vi "Configure Multi Eval Meas List Segment Modulation.vi"(0 "VISA resource name":refnum<visa-resource-name>, 1 "Enable (Off)":bool, 2 "MERR Enable (Off)":bool, 3 "Inband Emission Enable (Off)":bool, 5 "Instance (1)":T1=1, 7 "Segment (1)":i32=1, 9 "Statistics (20)":i32=20, 11 "error in (no error)":errorcluster, 12 "EVM Enable (Off)":bool, 13 "PERR Enable (Off)":bool, 14 "EQ Spectrum Flatness Enable (Off)":bool) -> (4 "VISA resource name out":refnum<visa-resource-name>, 15 "error out":errorcluster)   [LabVIEW 2020, in "Rohde&Schwarz CMWXP NR FR1 Measurement.lvlib"]
doc: "Defines settings for modulation measurements in list mode for segment <no>.\n\nAttribute:\nRSCMWXPNRFR1M_ATTR_MULTI_EVAL_MEAS_LIST_SEGMENT_MODULATION\n\nRemote-control command:\nCONFigure:NRSub:MEAS<i>:MEValuation:LIST:SEGMent<no>:MODulation"
uses:
  <instrlib>/Rohde&Schwarz CMWXP NR FR1 Measurement/Rohde&Schwarz CMWXP NR FR1 Measurement.lvlib
  <instrlib>/Rohde&Schwarz CMWXP NR FR1 Measurement/Private/_Instance.ctl
  <instrlib>/Rohde&Schwarz CMWXP NR FR1 Measurement/Private/rsidr_core.llb/rsidr_core.lvlib
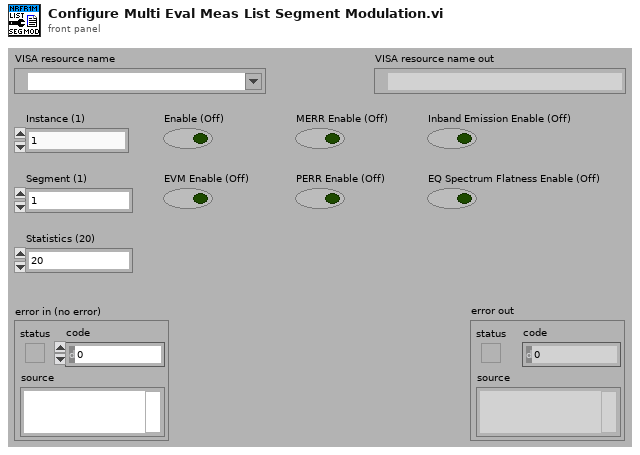
[diagram p1: front panel]
types:
  T1 = typedef "Rohde&Schwarz CMWXP NR FR1 Measurement.lvlib/_Instance.ctl" = i32
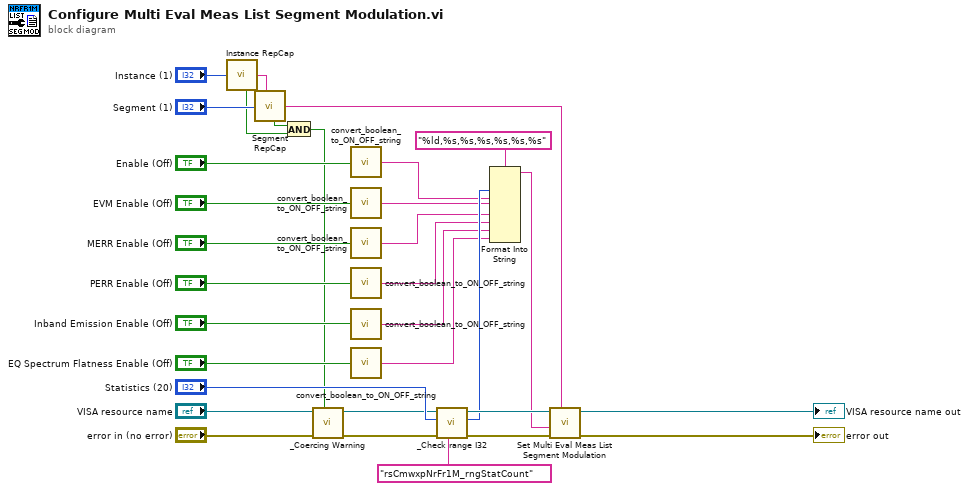
[diagram p0: block diagram]
diagram:
  n1 = call <instrlib>:"Instance RepCap.vi"("Instance In"="Instance (1)") -> ("In Range?"=w3:bool, "RepCap Identifier Out"=w18:string)  [unwired: 1 in]
  n2 = call <instrlib>:"Segment RepCap.vi"("Segment In"="Segment (1)", "RepCap String In (\"\")"=w18) -> ("In Range?"=w2:bool, "RepCap Identifier Out"=w17:string)
  n3 = And(x=w2, y=w3) -> (x .and. y?=w1:bool)
  n4 = call <instrlib>:"_Coercing Warning.vi"("In Range?"=w1, "error in (no error)"="error in (no error)", "VISA resource name"="VISA resource name") -> ("error out"=w5:errorcluster, "VISA resource name out"=w4:refnum<visa-resource-name>)  [unwired: 7 in]
  n5 = call <instrlib>:"convert_boolean_to_ON_OFF_string.vi"("boolean value in"="Enable (Off)") -> ("string value out"=w14:string)  [unwired: 4 in]
  n6 = call <instrlib>:"convert_boolean_to_ON_OFF_string.vi"("boolean value in"="EVM Enable (Off)") -> ("string value out"=w13:string)  [unwired: 4 in]
  n7 = call <instrlib>:"convert_boolean_to_ON_OFF_string.vi"("boolean value in"="MERR Enable (Off)") -> ("string value out"=w12:string)  [unwired: 4 in]
  n8 = call <instrlib>:"convert_boolean_to_ON_OFF_string.vi"("boolean value in"="PERR Enable (Off)") -> ("string value out"=w11:string)  [unwired: 4 in]
  n9 = call <instrlib>:"convert_boolean_to_ON_OFF_string.vi"("boolean value in"="Inband Emission Enable (Off)") -> ("string value out"=w10:string)  [unwired: 4 in]
  n10 = call <instrlib>:"convert_boolean_to_ON_OFF_string.vi"("boolean value in"="EQ Spectrum Flatness Enable (Off)") -> ("string value out"=w9:string)  [unwired: 4 in]
  n11 = call <instrlib>:"_Check range I32.vi"("Range Table Identifier"="rsCmwxpNrFr1M_rngStatCount", "error in (no error)"=w5, "I32 Value In"="Statistics (20)", "VISA resource name"=w4) -> ("error out"=w32:errorcluster, "I32 Value Out"=w15:i32, "VISA resource name out"=w29:refnum<visa-resource-name>)  [unwired: 5 in]
  n12 = Format Into String(format string="%ld,%s,%s,%s,%s,%s,%s", w15, w14, w13, w12, w11, w10, w9) -> (resulting string=w8:string)  [unwired: 2 in, 1 out]
  n13 = call "Set Multi Eval Meas List Segment Modulation"("Repeated Capabilities"=w17, "error in (no error)"=w32, "Multi Eval Meas List Segment Modulation ()"=w8, "instrument handle"=w29) -> ("error out"=→"error out":errorcluster, "instrument handle out"=→"VISA resource name out":refnum<visa-resource-name>)  [unwired: 6 in]
